vi "ProbabilityOfMissionSuccess.vi"(8 "Error In":errorcluster, 10 "MissionData":T1, 11 "B1 In":refnum<class "B1.lvclass">) -> (0 "Error out":errorcluster, 2 "Probability":dbl, 3 "B1 Out":refnum<class "B1.lvclass">)   [LabVIEW 2021, in "B1.lvclass"]
uses:
  B1.lvclass
  BattleDroid/BattleDroid.lvclass
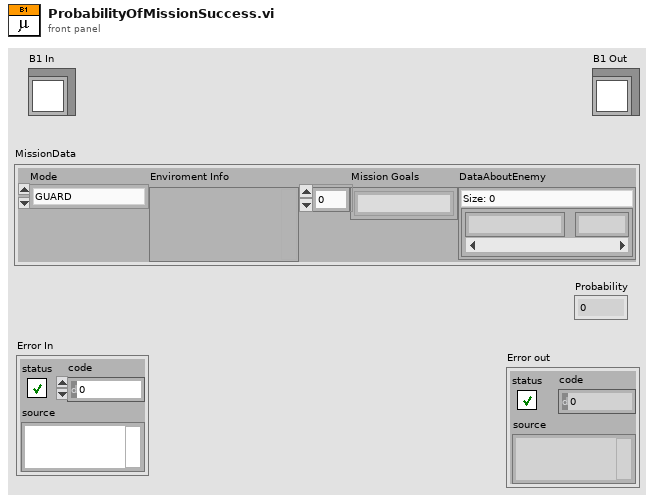
[diagram p1: front panel]
types:
  T1 = cluster{"Mode ":enum16{"GUARD", "RECON", "ATTACK ", "MAINTAINCE"}, "Enviroment Info":variant, "Mission Goals":string[], "DataAboutEnemy":map{string, i32}}
  T2 = enum16{"GUARD", "RECON", "ATTACK ", "MAINTAINCE"}
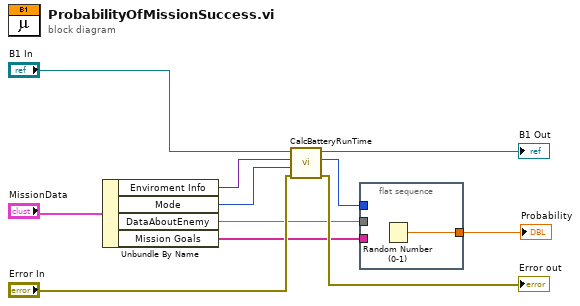
[diagram p0: block diagram]
diagram:
  n1 = Unbundle By Name("MissionData") -> ("Enviroment Info"=w6:variant, "Mode"=w5:T2, "DataAboutEnemy"=w3:map{string, i32}, "Mission Goals"=w2:string[])
  n2 = call "CalcBatteryRunTime.vi"("Error In"="Error In", "Mode"=w5, "Enviroment Info"=w6, "BattleDroid In"="B1 In") -> ("Error Out"=→"Error out":errorcluster, "Battery RunTime"=w4:u64, "BattleDroid Out"=→"B1 Out":refnum<class "B1.lvclass">)  [unwired: 5 in]
  n3 = flat-sequence {
    tunnel: w4 -> [_]
    tunnel: w3 -> [_]
    tunnel: w2 -> [_]
    tunnel: [w12] -> w1
    frame #0 {
      n4 = Random Number (0-1)() -> (number: 0 to 1=w12:dbl)
    }
  }
  "Probability" <- w1
